vi "GetMode.vi"(1 "Button":T1(ring)) -> (0 "Mode":enum16{"Default", "Toggle"}(ring))   [LabVIEW 2010, in "FTC.lvlib" / "Remote Interface.lvlib"]
uses:
  Remote Interface.lvlib
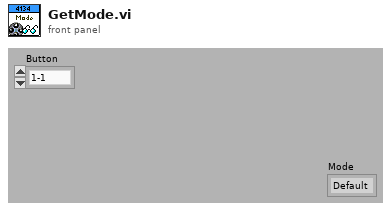
[diagram p1: front panel]
types:
  T1 = enum16{"1-1", "1-2", "1-3", "1-4", "1-5", "1-6", "1-7", "1-8", "1-9", "1-10", "1-11", "1-12", "2-1", "2-2", "2-3", "2-4", "2-5", "2-6", "2-7", "2-8", "2-9", "2-10", "2-11", "2-12", "NXT-L", "NXT-R", "NXT-E", "1-U", "1-UR", "1-R", "1-DR", "1-D", "1-DL", "1-L", "1-UL", "2-U", "2-UR", "2-R", "2-DR", "2-D", "2-DL", "2-L", "2-UL"}
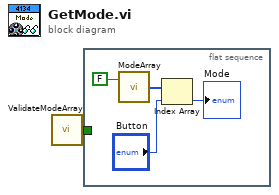
[diagram p0: block diagram]
diagram:
  n1 = call "ValidateModeArray.vi"() -> ("Valid?"=w1:bool)
  n2 = flat-sequence {
    tunnel: w1 -> [_]
    frame #0 {
      n3 = call "ModeArray.vi"("Write?"=FALSE) -> ("Array"=w4:u16[])  [unwired: 1 in]
      n4 = Index Array(array=w4, index="Button") -> (element=→"Mode":u16)
    }
  }
